vi "Cal Inst Control.vi"(8 "error in (no error)":errorcluster, 10 "Master":refnum<queue>, 11 "Sub Panel ref":refnum<vi>) -> (0 "error out":errorcluster)   [LabVIEW 2013]
uses:
  CaliforniaInstrumentsIxSeries/support/Message Queue/Message Cluster.ctl
  CaliforniaInstrumentsIxSeries/support/Message Queue/Cal Inst Message Queue.lvlib
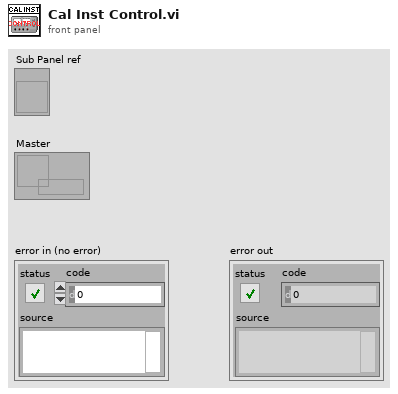
[diagram p1: front panel]
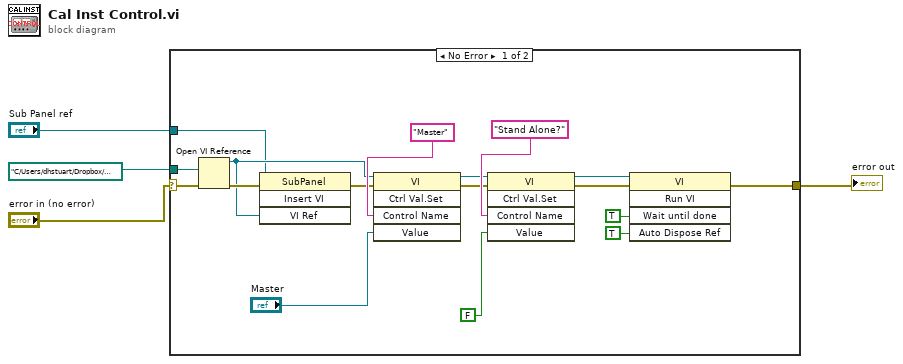
[diagram p0: block diagram]
diagram:
  n1 = case shown="No Error" "error in (no error)" {
    selector: "error in (no error)" -> [w5 w22]
    tunnel: [w13 w22] -> w4
    tunnel: path "C:/Users/dhstuart/Dropbox/CLTC/CaliforniaInstrumentsIxSeries/Cal Inst Main.vi" -> [w11 _]
    tunnel: "Sub Panel ref" -> [w8 _]
    frame No Error {
      n2 = Open VI Reference(vi path=w11, error in (no error)=w5) -> (vi reference=w9:refnum<vi>, error out=w12:errorcluster)  [unwired: 4 in]
      n3 = invoke on="Invoke Node" class="SubPanel" method="Insert VI"(reference=w8, error in=w12, "VI Ref"=w9) -> (error out=w10:errorcluster)  [unwired: 1 in, 3 out]
      n4 = invoke class="VI" method="Ctrl Val.Set"(reference=w9, error in=w10, "Control Name"="Master", "Value"="Master") -> (reference out=w7:refnum<vi>, error out=w6:errorcluster)  [unwired: 1 in, 3 out]
      n5 = invoke class="VI" method="Ctrl Val.Set"(reference=w7, error in=w6, "Control Name"="Stand Alone?", "Value"=FALSE) -> (reference out=w17:refnum<vi>, error out=w16:errorcluster)  [unwired: 1 in, 3 out]
      n6 = invoke class="VI" method="Run VI"(reference=w17, error in=w16, "Wait until done"=TRUE ("Wait Until Done"), "Auto Dispose Ref"=TRUE ("Auto Dispose Reference")) -> (error out=w13:errorcluster)  [unwired: 1 in, 4 out]
    }
    frame Error {
    }
  }
  "error out" <- w4
